vi "LEM_V2.vi"() -> ()   [LabVIEW 2012]
uses:
  Model.ctl
  Utilities/fluid_properties/fluid_types.ctl
  <vilib>/Simulation/Implementation/Shared/SIM Continuous Solvers.ctl
  LEM_States.ctl
  SJ_ODE_Data.ctl
  Utilities/fluid_properties/fluid_properties.ctl
  <vilib>/Simulation/Utility/Implementation/Shared/SIM Diagram Parameters.ctl
  <vilib>/Analysis/1siggen.llb/Ramp Pattern by Samples.vi
  <vilib>/Analysis/baseanly.llb/Scale 1D.vi
  <vilib>/Analysis/NI_AALBase.lvlib
  <vilib>/Analysis/NI_AALPro.lvlib
panel:
  out "Start":u32
  in  "Tab Control":T1(tab)
  in  "Fluid Properties":T3={"Fluid"=enum."Air", "Temperature (K)"=295.0, "Pressure (Pa)"=101325.0}
  in  "Solution Controls":T5={"Simulation"=enum."Sinusoidal", "Fixed Parameter"=enum."Displacement", "Model"=enum."Tang", "# time steps"=50, "# periods"=500, "Domain"=enum."Time", "Tolerance"=1e-08, "STFT periods"=5}
  in  "Forcing Functiuon":T6={"Fixed Parameter Amp"=5e-05, "type"=0, "Start Frequency"=335.0, "Stop Frequency"=1340.0, "# frequency steps"=100} {"type" items=["Linear", "Logarithmic"]}
  in  "SJ Geometry":T7={"Do (mm)"=5.0, "Ho (mm)"=9.0, "Dc (mm)"=40.0, "Hc (mm)"=9.0}
  in  "Continuous Solver":T8=enum."Runge-Kutta 4"
  out "Trajectory":cluster{dbl[], dbl[]}(graph)
  out "Convergence":cluster{dbl[], dbl[]}(graph)
  out "Time Trace":cluster{dbl[], dbl[]}(graph)
  in  "Plot Data?":bool
  out "|Uo|":cluster{"Ramp Pattern":dbl[], dbl[]}(graph)
  out "Phase Angle":cluster{"Ramp Pattern":dbl[], dbl[]}(graph)
  out "Periods":cluster{"Ramp Pattern":dbl[], dbl[]}(graph)
  in  "Plot Data Coniuously?":bool
  out "Model Runtime (ms)":u32
  out "f_H":dbl
  # "Use only fixed step solvers!"
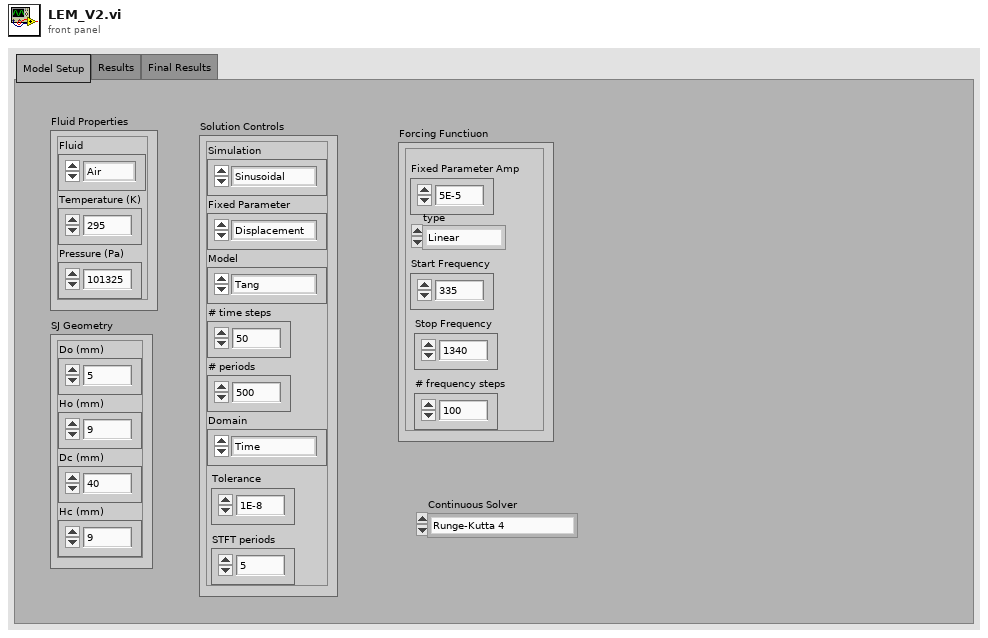
[diagram p1: front panel]
types:
  T1 = enum32{"Model Setup", "Results", "Final Results"}
  T2 = typedef "fluid_types.ctl" = enum16{"Air", "Water"}
  T3 = cluster{"Fluid":T2, "Temperature (K)":dbl, "Pressure (Pa)":dbl}
  T4 = typedef "Model.ctl" = enum16{"Tang", "Gallas", "Persoon"}
  T5 = cluster{"Simulation":enum16{"Asymmetric", "Sinusoidal"}, "Fixed Parameter":enum16{"Pressure", "Displacement"}, "Model":T4, "# time steps":i32, "# periods":i32, "Domain":enum16{"Time", "Frequency"}, "Tolerance":dbl, "STFT periods":i32}
  T6 = cluster{"Fixed Parameter Amp":dbl, "type":u16, "Start Frequency":dbl, "Stop Frequency":dbl, "# frequency steps":i32}
  T7 = cluster{"Do (mm)":dbl, "Ho (mm)":dbl, "Dc (mm)":dbl, "Hc (mm)":dbl}
  T8 = typedef "SIM Continuous Solvers.ctl" = enum16{"Runge-Kutta 1 (Euler)", "Runge-Kutta 2", "Runge-Kutta 3", "Runge-Kutta 4", "Runge-Kutta 23 (variable)", "Runge-Kutta 45 (variable)", "BDF (variable)", "Adams-Moulton (variable)", "Rosenbrock (variable)", "Discrete States Only"}
  T9 = typedef "LEM_States.ctl" = enum16{"Setup_Model", "End", "Next_Frequency", "Solve_Model", "Convergence_Check"}
  T10 = typedef "SIM Diagram Parameters.ctl" = cluster{"Initial Time":dbl, "Final Time":dbl, "Time Step":dbl, "Absolute Tolerance":dbl, "Relative Tolerance":dbl, "Continuous Solver":T8, "Discrete Time Step":dbl, "Minimum Time Step":dbl, "Maximum Time Step":dbl, "Initial Time Step":dbl}
  T11 = typedef "SJ_ODE_Data.ctl" = cluster{"Fluid Properties":cluster{"Fluid":T2, "Temperature (K)":dbl, "Pressure (Pa)":dbl}, "SJ Geometry":cluster{"Do (mm)":dbl, "Ho (mm)":dbl, "Dc (mm)":dbl, "Hc (mm)":dbl}, "Solution Controls":cluster{"Simulation":enum16{"Asymmetric", "Sinusoidal"}, "Fixed Parameter":enum16{"Pressure", "Displacement"}, "Model":T4, "# time steps":i32, "# periods":i32, "Domain":enum16{"Time", "Frequency"}, "Tolerance":dbl, "STFT periods":i32}, "Misc Data":cluster{"Amplitude Array":dbl[], "Freq jet":dbl, "Coefficients":dbl[], "Nat Frequ":dbl}, "Thermo and Transport Properties":T12, "LEM Output Data":cluster{"X":dbl[][], "times":dbl[], "|X|":dbl, "PA X":dbl}}
  T12 = typedef "fluid_properties.ctl" = cluster{"nu":dbl, "c":dbl, "Pr":dbl, "Cp":dbl, "Cv":dbl, "gamma":dbl, "mu":dbl, "rho":dbl}
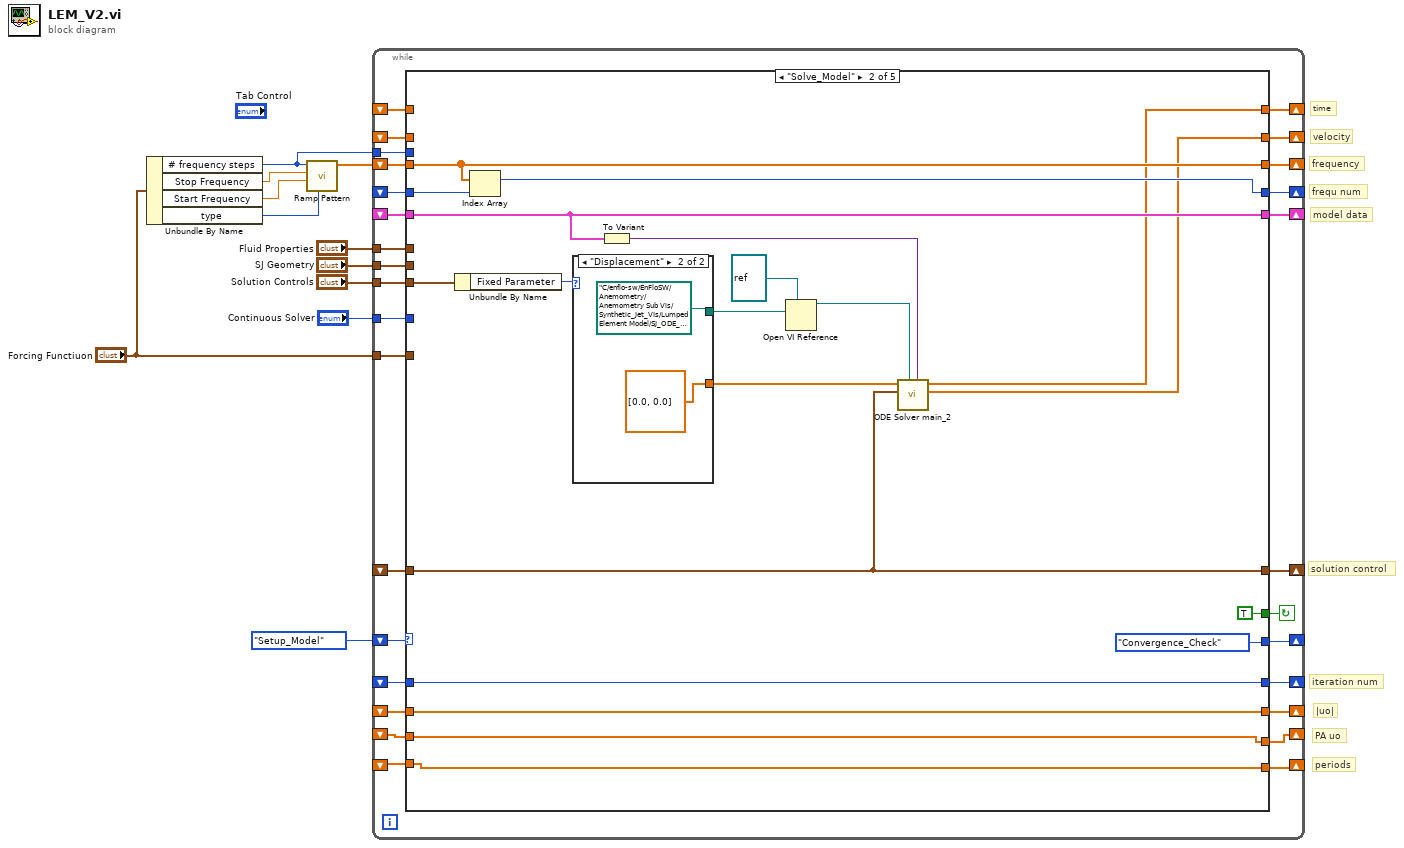
[diagram p0: block diagram]
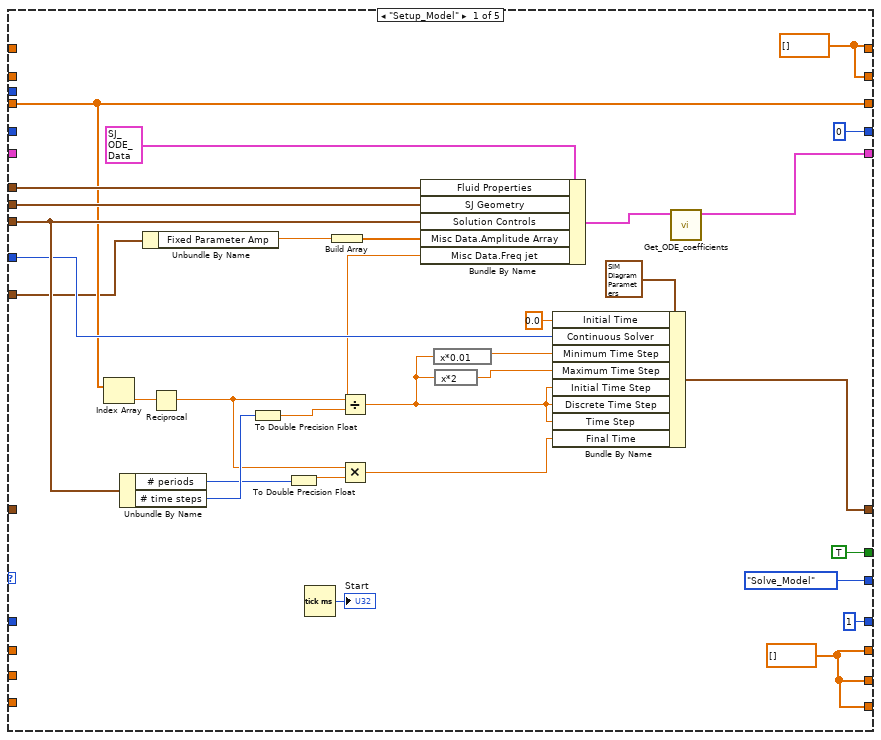
[diagram p2: hidden frame]
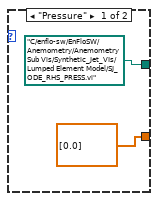
[diagram p3: hidden frame]
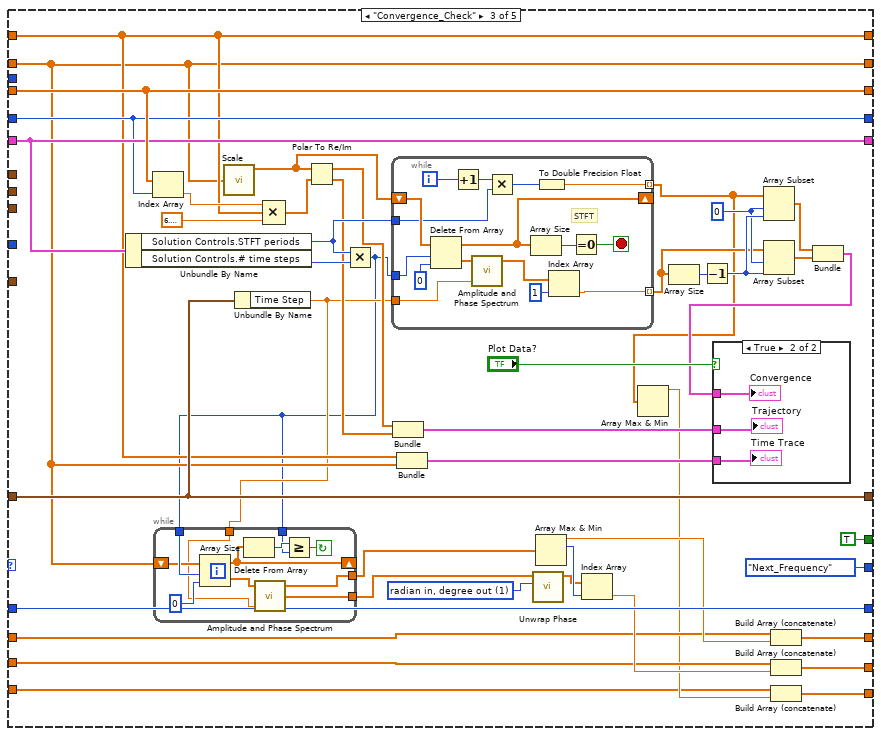
[diagram p4: hidden frame]
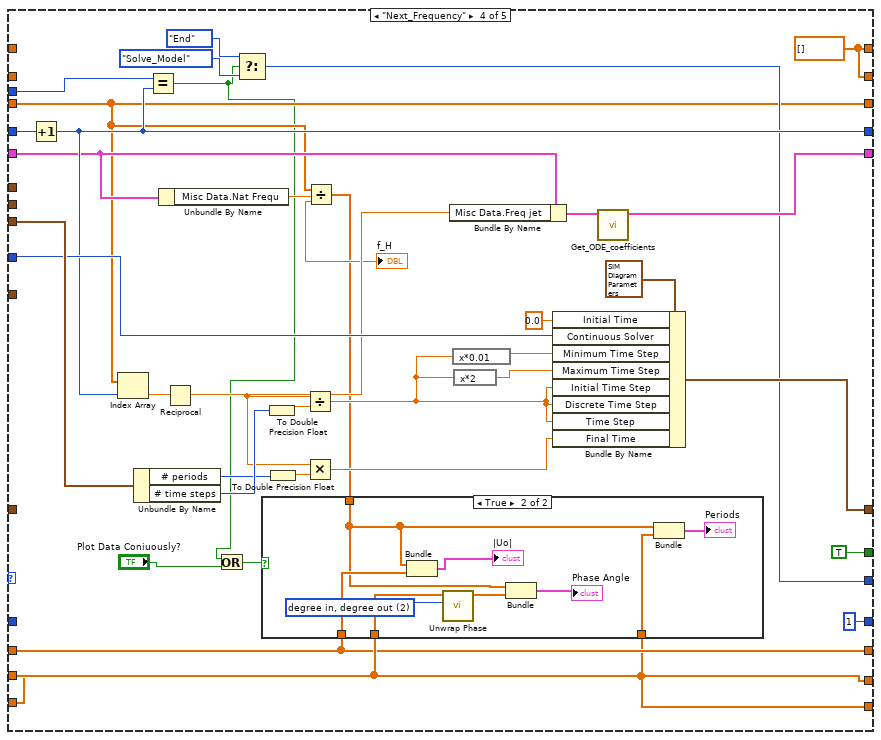
[diagram p6: hidden frame]
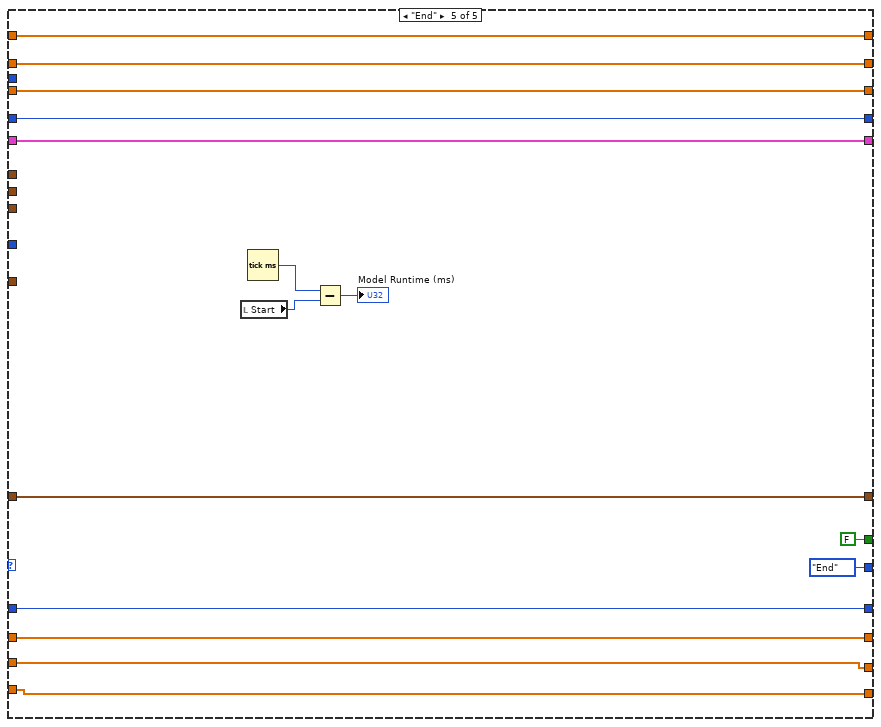
[diagram p8: hidden frame]
diagram:
  # "periods"
  # "PA uo"
  # "|uo|"
  # "iteration num"
  # "solution control"
  # "model data"
  # "frequ num"
  # "frequency"
  # "velocity"
  # "time"
  n1 = Unbundle By Name("Forcing Functiuon") -> ("# frequency steps"=w1:i32, "Stop Frequency"=w5:dbl, "Start Frequency"=w6:dbl, "type"=w7:u16)
  n2 = call-poly <vilib>:"Ramp Pattern.vi"("type"=w7, "start"=w6, "end"=w5, "samples"=w1) -> ("Ramp Pattern"=w4:dbl[])  [unwired: 6 in, 1 out]
  n3 = while {
    tunnel: "Fluid Properties" -> [w39]
    tunnel: "SJ Geometry" -> [w38]
    tunnel: "Solution Controls" -> [w37]
    shift-right: [w36] -> _
    shift-left: _ -> [w35]
    tunnel: "Forcing Functiuon" -> [w34]
    shift-right: [w32] -> _
    shift-left: _ -> [w33]
    shift-right: [w30] -> _
    shift-left: w4 -> [w31]
    shift-right: [w22] -> _
    shift-left: LEM_States."Setup_Model" -> [w29]
    shift-right: [w28] -> _
    shift-left: _ -> [w27]
    tunnel: "Continuous Solver" -> [w26]
    shift-right: [w14] -> _
    shift-left: _ -> [w25]
    shift-right: [w24] -> _
    shift-left: _ -> [w23]
    shift-right: [w21] -> _
    shift-left: _ -> [w20]
    tunnel: w1 -> [w19]
    shift-right: [w18] -> _
    shift-left: _ -> [w16]
    shift-right: [w17] -> _
    shift-left: _ -> [w15]
    shift-right: [w13] -> _
    shift-left: _ -> [w12]
    stop <- w40 continue-if-true
    n4 = case shown="\"Solve_Model\"" w29 {
      tunnel: [TRUE TRUE TRUE TRUE FALSE] -> w40
      tunnel: w39 -> [w69 _ _ _ _]
      tunnel: w38 -> [w68 _ _ _ _]
      tunnel: w37 -> [w64 w86 _ w201 _]
      tunnel: [w66 w84 w133 w202 w224] -> w36
      tunnel: w35 -> [_ w84 w133 w175 w224]
      tunnel: w34 -> [w47 _ _ _ _]
      tunnel: w33 -> [_ w88 w129 w196 w225]
      tunnel: [0 w88 w129 w183 w225] -> w32
      tunnel: w31 -> [w59 w89 w136 w173 w226]
      tunnel: [w59 w89 w136 w173 w226] -> w30
      tunnel: [w63 w76 w130 w200 w223] -> w28
      tunnel: w27 -> [_ w76 w130 _ w223]
      tunnel: w26 -> [w61 _ _ w198 _]
      tunnel: [w43 w72 w103 w177 w227] -> w14
      tunnel: w25 -> [_ _ w103 _ w227]
      tunnel: [w43 w73 w124 w177 w228] -> w24
      tunnel: w23 -> [_ _ w124 _ w228]
      tunnel: [LEM_States."Solve_Model" LEM_States."Convergence_Check" LEM_States."Next_Frequency" w180 LEM_States."End"] -> w22
      tunnel: [1 w81 w122 1 w222] -> w21
      tunnel: w20 -> [_ w81 w122 _ w222]
      tunnel: w19 -> [_ _ _ w184 _]
      tunnel: [w42 w80 w116 w178 w219] -> w18
      tunnel: [w42 w79 w98 w179 w218] -> w17
      tunnel: w16 -> [_ w80 w115 w178 w219]
      tunnel: w15 -> [_ w79 w114 w179 w218]
      tunnel: [w42 w78 w97 w176 w217] -> w13
      tunnel: w12 -> [_ w78 w95 w176 w217]
      frame "Setup_Model" {
        w42 = dbl[] []
        w43 = dbl[] []
        n5 = Index Array(array=w59) -> (element=w48:dbl)  [unwired: 1 in]
        n6 = Unbundle By Name(w64) -> ("# periods"=w54:i32, "# time steps"=w58:i32)
        n7 = Unbundle By Name(w47) -> ("Fixed Parameter Amp"=w46:dbl)
        n8 = Reciprocal(x=w48) -> (1/x=w52:dbl)
        n9 = To Double Precision Float(number=w58) -> (double precision float=w57:dbl)
        n10 = To Double Precision Float(number=w54) -> (double precision float=w53:dbl)
        n11 = Tick Count (ms)() -> (millisecond timer value=→"Start":u32)
        n12 = Build Array(w46) -> (w45:dbl[])
        n13 = Divide(x=w52, y=w57) -> (x/y=w50:dbl)
        n14 = Multiply(x=w52, y=w53) -> (x*y=w51:dbl)
        n15 = Bundle By Name(cluster=T11 {"Fluid Properties"={"Fluid"=enum."Air", "Temperature (K)"=300.0, "Pressure (Pa)"=100000.0}, "SJ Geometry"={"Do (mm)"=5.0, "Ho (mm)"=8.0, "Dc (mm)"=40.0, "Hc (mm)"=6.5}, "Solution Controls"={"Simulation"=enum."Asymmetric", "Fixed Parameter"=enum."Pressure", "Model"=enum."Tang", "# time steps"=1, "# periods"=340, "Domain"=enum."Time", "Tolerance"=0.0, "STFT periods"=0}, "Misc Data"={"Amplitude Array"=[], "Freq jet"=1.205, "Coefficients"=[], "Nat Frequ"=0.0}, "Thermo and Transport Properties"={"nu"=0.0, "c"=0.0, "Pr"=0.0, "Cp"=0.0, "Cv"=0.0, "gamma"=0.0, "mu"=0.0, "rho"=0.0}, "LEM Output Data"={"X"=[], "times"=[], "|X|"=0.0, "PA X"=0.0}} ("ODE Data"), "Fluid Properties"=w69, "SJ Geometry"=w68, "Solution Controls"=w64, "Misc Data.Amplitude Array"=w45, "Misc Data.Freq jet"=w48) -> (w70:T11)
        n16 = expression code="x*0.01"(w50) -> (w55:dbl)
        n17 = expression code="x*2"(w50) -> (w56:dbl)
        n18 = Bundle By Name(cluster=T10 {"Initial Time"=0.0, "Final Time"=10.0, "Time Step"=0.1, "Absolute Tolerance"=0.001, "Relative Tolerance"=0.001, "Continuous Solver"=enum."Runge-Kutta 45 (variable)", "Discrete Time Step"=1.0, "Minimum Time Step"=1e-08, "Maximum Time Step"=1.0, "Initial Time Step"=0.01} ("simulation parameters"), "Initial Time"=0.0, "Continuous Solver"=w61, "Minimum Time Step"=w55, "Maximum Time Step"=w56, "Initial Time Step"=w50, "Discrete Time Step"=w50, "Time Step"=w50, "Final Time"=w51) -> (w63:T10)
        n19 = call "Get_ODE_coefficients.vi"("ODE Data in"=w70) -> ("ODE Data out"=w66:T11)  [unwired: 10 in]
      }
      frame "Solve_Model" {
        n20 = Unbundle By Name(w86) -> ("Fixed Parameter"=w83:enum16{"Pressure", "Displacement"})
        n21 = Index Array(array=w89, index=w88) -> ()  [unwired: 1 out]
        n22 = case shown="\"Displacement\"" w83 {
          tunnel: [path "C:/enflo-sw/EnFloSW/Anemometry/Anemometry Sub Vis/Synthetic_Jet_VIs/Lumped Element Model/SJ_ODE_RHS_PRESS.vi" ("vi path") path "C:/enflo-sw/EnFloSW/Anemometry/Anemometry Sub Vis/Synthetic_Jet_VIs/Lumped Element Model/SJ_ODE_RHS_DISP.vi" ("vi path")] -> w85
          tunnel: [dbl[] [0.0] ("x0") dbl[] [0.0, 0.0] ("x0")] -> w77
          frame "Pressure" {
          }
          frame "Displacement" {
          }
        }
        n23 = To Variant(anything=w84) -> (Variant=w74:variant)
        n24 = Open VI Reference(type specifier VI Refnum (for type only)=refnum<vi> refnum, vi path=w85) -> (vi reference=w75:refnum<vi>)  [unwired: 4 in, 1 out]
        n25 = call <vilib>:"ODE Solver main_2.vi"("data"=w74, "ODE F(X,t)"=w75, "simulation parameters"=w76, "x0"=w77) -> ("output"=w72:dbl[], "times"=w73:dbl[])  [unwired: 5 in, 1 out]
      }
      frame "Convergence_Check" {
        w119 = 1 items=["radian in, radian out", "radian in, degree out", "degree in, degree out", "degree in, radian out"] ("phase unit")
        w109 = 0 ("index")
        n26 = Unbundle By Name(w133) -> ("Solution Controls.STFT periods"=w132:i32, "Solution Controls.# time steps"=w131:i32)
        n27 = Index Array(array=w136, index=w129) -> (element=w135:dbl)
        n28 = call-poly <vilib>:"Scale.vi"("X"=w103) -> ("Y=(X-offset)/scale"=w105:dbl[])  [unwired: 3 out]
        n29 = Unbundle By Name(w130) -> ("Time Step"=w101:dbl)
        n30 = Compound Arithmetic op=MULTIPLY(w135, w124, 6.283185307179586) -> (w134:dbl[])
        n31 = Polar To Re/Im(2:w134, 3:w105) -> (0:w126:dbl[], 1:w104:dbl[])
        n32 = Multiply(x=w132, y=w131) -> (x*y=w100:i32)
        n33 = while {
          tunnel: w100 -> [w148]
          shift-right: [w145] -> _
          shift-left: w103 -> [w147]
          tunnel: [w144] -> w112
          tunnel: [w143] -> w113
          tunnel: w101 -> [w142]
          tunnel: w100 -> [w139]
          stop <- w141 continue-if-true
          n34 = Delete From Array(array=w147, length=w148, index=0) -> (deleted portion=w146:dbl[], array with subset deleted=w145:dbl[])
          n35 = Array Size(array=w145) -> (size(s)=w140:i32)
          n36 = call <vilib>:"Amplitude and Phase Spectrum.vi"("dt"=w142, "Signal (V)"=w146) -> ("Amp Spectrum Phase (radians)"=w143:dbl[], "Amp Spectrum Mag (Vrms)"=w144:dbl[])  [unwired: 1 in, 1 out]
          n37 = Greater Or Equal?(x=w140, y=w139) -> (x >= y?=w141:bool)
        }
        n38 = while {
          tunnel: w101 -> [w168]
          shift-right: [w164] -> _
          shift-left: w105 -> [w165]
          tunnel: w100 -> [w166]
          tunnel: [w153] -> w102 mode=indexing
          tunnel: [w159] -> w99 mode=indexing
          tunnel: w132 -> [w156]
          i -> [w158]
          stop <- w162 stop-if-true
          # "STFT"
          n39 = Delete From Array(array=w165, length=w166, index=0) -> (deleted portion=w161:dbl[], array with subset deleted=w164:dbl[])
          n40 = Increment(x=w158) -> (x+1=w157:i32)
          n41 = call <vilib>:"Amplitude and Phase Spectrum.vi"("dt"=w168, "Signal (V)"=w161) -> ("Amp Spectrum Mag (Vrms)"=w154:dbl[])  [unwired: 1 in, 2 out]
          n42 = Multiply(x=w157, y=w156) -> (x*y=w155:i32)
          n43 = Array Size(array=w164) -> (size(s)=w163:i32)
          n44 = To Double Precision Float(number=w155) -> (double precision float=w159:dbl)
          n45 = Index Array(array=w154, index=1) -> (element=w153:dbl)
          n46 = Equal To 0?(x=w163) -> (x = 0?=w162:bool)
        }
        n47 = Bundle(w104, w126) -> (w125:cluster{dbl[], dbl[]})  [unwired: 1 in]
        n48 = Bundle("times"=w124, "output"=w103) -> (w123:cluster{"times":dbl[], "output":dbl[]})  [unwired: 1 in]
        n49 = call <vilib>:"Unwrap Phase.vi"("phase unit"=w119, "Phase"=w113) -> ("Unwrapped Phase"=w120:dbl[])  [unwired: 8 in, 1 out]
        n50 = Array Max & Min(array=w112) -> (max value=w118:dbl, max index (indices)=w121:i32)  [unwired: 2 out]
        n51 = Index Array(array=w120, index=w121) -> (element=w117:dbl)
        n52 = Array Max & Min(array=w99) -> (max value=w96:dbl)  [unwired: 3 out]
        n53 = Array Size(array=w102) -> (size(s)=w107:i32)
        n54 = Decrement(x=w107) -> (x-1=w110:i32)
        n55 = Array Subset(array=w99, index=w109, length=w110) -> (w111:dbl[])
        n56 = Array Subset(array=w102, index=w109, length=w110) -> (w108:dbl[])
        n57 = Build Array (concatenate)(w115, w118) -> (w116:dbl[])
        n58 = Build Array (concatenate)(w114, w117) -> (w98:dbl[])
        n59 = Build Array (concatenate)(w95, w96) -> (w97:dbl[])
        n60 = Bundle(w111, w108) -> (w127:cluster{dbl[], dbl[]})  [unwired: 1 in]
        n61 = case shown="True" "Plot Data?" {
          tunnel: w127 -> [_ w152]
          tunnel: w125 -> [_ w151]
          tunnel: w123 -> [_ w150]
          frame False {
          }
          frame True {
            "Convergence" <- w152
            "Trajectory" <- w151
            "Time Trace" <- w150
          }
        }
      }
      frame "Next_Frequency" {
        w177 = dbl[] []
        n62 = Increment(x=w196) -> (x+1=w183:i32)
        n63 = Index Array(array=w173, index=w183) -> (element=w186:dbl)
        n64 = Unbundle By Name(w201) -> ("# periods"=w191:i32, "# time steps"=w195:i32)
        n65 = Equal?(x=w184, y=w183) -> (x = y?=w170:bool)
        n66 = Unbundle By Name(w175) -> ("Misc Data.Nat Frequ"=w174:dbl)
        "f_H" <- w174
        n67 = Reciprocal(x=w186) -> (1/x=w189:dbl)
        n68 = Or(x=w170, y="Plot Data Coniuously?") -> (x .or. y?=w169:bool)
        n69 = Select(t=LEM_States."End", s=w170, f=LEM_States."Solve_Model") -> (s? t:f=w180:T9)
        n70 = To Double Precision Float(number=w195) -> (double precision float=w194:dbl)
        n71 = To Double Precision Float(number=w191) -> (double precision float=w190:dbl)
        n72 = Divide(x=w189, y=w194) -> (x/y=w187:dbl)
        n73 = Multiply(x=w189, y=w190) -> (x*y=w188:dbl)
        n74 = Divide(x=w173, y=w174) -> (x/y=w172:dbl[])
        n75 = case shown="True" w169 {
          tunnel: w179 -> [_ w213]
          tunnel: w178 -> [_ w212]
          tunnel: w176 -> [_ w206]
          tunnel: w172 -> [_ w205]
          frame False {
          }
          frame True {
            w208 = 2 items=["radian in, radian out", "radian in, degree out", "degree in, degree out", "degree in, radian out"] ("phase unit")
            n76 = Bundle(w205, w212) -> (→"|Uo|":cluster{dbl[], dbl[]})  [unwired: 1 in]
            n77 = call <vilib>:"Unwrap Phase.vi"("phase unit"=w208, "Phase"=w213) -> ("Unwrapped Phase"=w209:dbl[])  [unwired: 8 in, 1 out]
            n78 = Bundle(w205, "Unwrapped Phase"=w209) -> (→"Phase Angle":cluster{dbl[], "Unwrapped Phase":dbl[]})  [unwired: 1 in]
            n79 = Bundle(w205, w206) -> (→"Periods":cluster{dbl[], dbl[]})  [unwired: 1 in]
          }
        }
        n80 = Bundle By Name(cluster=w175, "Misc Data.Freq jet"=w186) -> (w203:T11)
        n81 = expression code="x*0.01"(w187) -> (w192:dbl)
        n82 = expression code="x*2"(w187) -> (w193:dbl)
        n83 = Bundle By Name(cluster=T10 {"Initial Time"=0.0, "Final Time"=10.0, "Time Step"=0.1, "Absolute Tolerance"=0.001, "Relative Tolerance"=0.001, "Continuous Solver"=enum."Runge-Kutta 45 (variable)", "Discrete Time Step"=1.0, "Minimum Time Step"=1e-08, "Maximum Time Step"=1.0, "Initial Time Step"=0.01} ("simulation parameters"), "Initial Time"=0.0, "Continuous Solver"=w198, "Minimum Time Step"=w192, "Maximum Time Step"=w193, "Initial Time Step"=w187, "Discrete Time Step"=w187, "Time Step"=w187, "Final Time"=w188) -> (w200:T10)
        n84 = call "Get_ODE_coefficients.vi"("ODE Data in"=w203) -> ("ODE Data out"=w202:T11)  [unwired: 10 in]
      }
      frame "End" {
        n85 = local read "Start"() -> (w216:u32)
        n86 = Tick Count (ms)() -> (millisecond timer value=w215:u32)
        n87 = Subtract(x=w215, y=w216) -> (x-y=→"Model Runtime (ms)":u32)
      }
    }
  }
